vi "StringClearZero.vi"(11 "String in":string) -> (3 "String out":string)   [LabVIEW 2017]
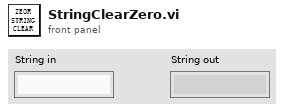
[diagram p1: front panel]
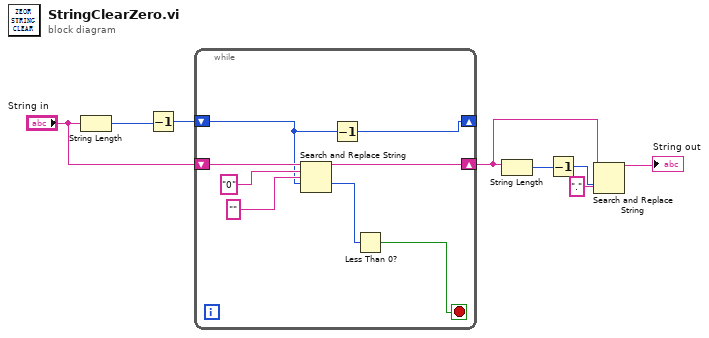
[diagram p0: block diagram]
diagram:
  n1 = String Length(string="String in") -> (length=w7:i32)
  n2 = Decrement(x=w7) -> (x-1=w6:i32)
  n3 = while {
    shift-right: [w9] -> _
    shift-left: w6 -> [w10]
    shift-right: [w13] -> w3
    shift-left: "String in" -> [w16]
    stop <- w11 stop-if-true
    n4 = Search and Replace String(input string=w16, search string="0", replace string="" ("replace string (\"\")"), offset=w10) -> (result string=w13:string, offset past replacement=w12:i32)  [unwired: 4 in, 2 out]
    n5 = Decrement(x=w10) -> (x-1=w9:i32)
    n6 = Less Than 0?(x=w12) -> (x < 0?=w11:bool)
  }
  n7 = String Length(string=w3) -> (length=w5:i32)
  n8 = Decrement(x=w5) -> (x-1=w4:i32)
  n9 = Search and Replace String(input string=w3, search string=".", offset=w4) -> (result string=→"String out":string)  [unwired: 5 in, 3 out]
